vi "Poll Until Idle.vi"(8 "error in (no error)":errorcluster, 9 "Device and Axis":string, 11 "VISA resource name":refnum<visa-resource-name>) -> (0 "error out":errorcluster, 3 "VISA resource name out":refnum<visa-resource-name>)   [LabVIEW 2018, in "Zaber A Series.lvlib"]
doc: "Waits for any movement of the device to complete and the device to be idle before continuing. To poll a specific device, use the Device and Axis input. This VI is not designed to poll all devices unless only one device is connected.\n\nTo avoid saturating the CPU or the communication channel, this VI will poll once every 25ms. There is no wait if the device is in the idle state.\n\nThis VI requires that the Initialize VI has been called with the same serial port."
uses:
  Zaber A Series.lvlib
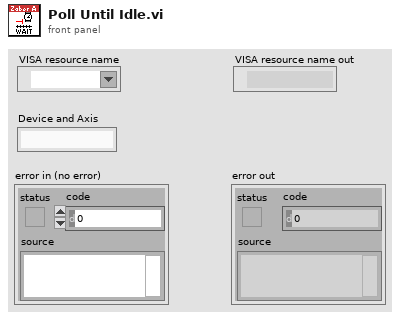
[diagram p1: front panel]
types:
  T1 = cluster{"Device":string, "Axis":string, "Reply Flag":string, "Status":string, "Warning Flags":string, "Data":string}[]
  T2 = cluster{"Device":string, "Axis":string, "Reply Flag":string, "Status":string, "Warning Flags":string, "Data":string}
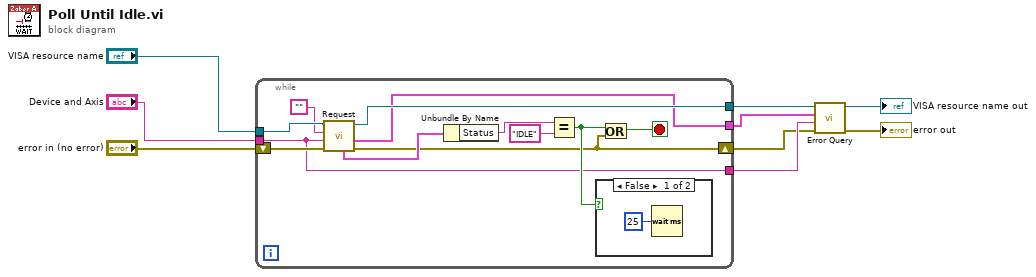
[diagram p0: block diagram]
diagram:
  n1 = while {
    tunnel: "VISA resource name" -> [w18]
    tunnel: [w17] -> w4
    tunnel: "Device and Axis" -> [w14]
    shift-right: [w10] -> w2
    shift-left: "error in (no error)" -> [w16]
    tunnel: [w12] -> w5
    tunnel: [w14] -> w6
    stop <- w11 stop-if-true
    n2 = call "Request.vi"("error in (no error)"=w16, "Device and Axis"=w14, "Command String"="", "VISA resource name"=w18) -> ("error out"=w10:errorcluster, "Response Bundle Array"=w12:T1, "VISA resource name out"=w17:refnum<visa-resource-name>, "First Response Bundle"=w13:T2)  [unwired: 2 in, 2 out]
    n3 = Unbundle By Name(w13) -> ("Status"=w20:string)
    n4 = Equal?(x=w20, y="IDLE") -> (x = y?=w19:bool)
    n5 = case shown="False" w19 {
      frame False {
        n6 = Wait (ms)(milliseconds to wait=u32 25) -> ()  [unwired: 1 out]
      }
      frame True {
      }
    }
    n7 = Or(x=w19, y=w10) -> (x .or. y?=w11:bool)
  }
  n8 = call "Error Query.vi"("error in (no error)"=w2, "Device and Axis"=w6, "Previous Response Bundle Array"=w5, "VISA resource name"=w4) -> ("error out"=→"error out":errorcluster, "VISA resource name out"=→"VISA resource name out":refnum<visa-resource-name>)  [unwired: 4 in, 2 out]
